vi "DAQmx Create Channel (TEDS-AI-Position-LVDT).vi"(0 "task in":refnum<k21>, 1 "maximum value":dbl=0.1 format="%0.2f", 2 "minimum value":dbl=-0.1 format="%0.2f", 3 "voltage excitation wire mode":i32(ring)=4 items=["4-Wire"=4, "5-Wire"=5, "6-Wire"=6], 5 "physical channels":tag, 6 "voltage excitation source":i32(ring)=10200 items=["Internal"=10200, "External"=10167, "None"=10230], 7 "name to assign":string, 8 "voltage excitation value":dbl=1.0, 9 "units":i32(ring)=10219 items=["Meters"=10219, "Inches"=10379, "From Custom Scale"=10065], 10 "voltage excitation frequency":dbl=2500.0, 11 "error in":errorcluster, 12 "custom scale name":tag) -> (4 "task out":refnum<k21>, 15 "error out":errorcluster)   [LabVIEW 2020]
doc: "Creates channel(s) that use an LVDT to measure linear position. You must configure the physical channel(s) with TEDS information to use this VI."
uses:
  nilvaiu.dll
panel:
  # "input limits"
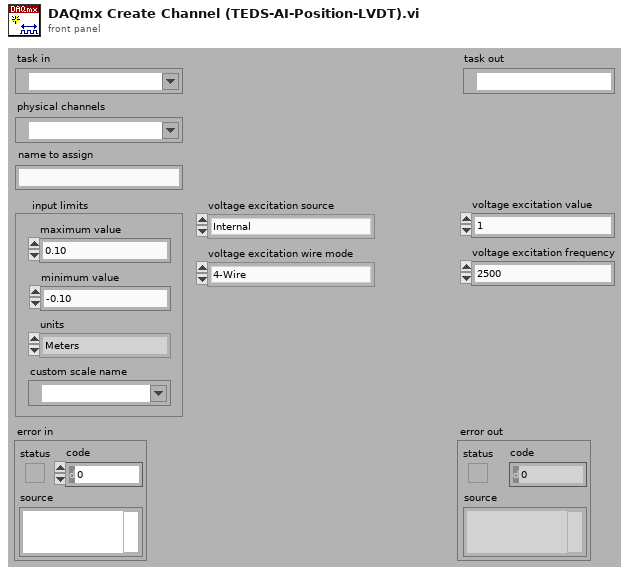
[diagram p1: front panel]
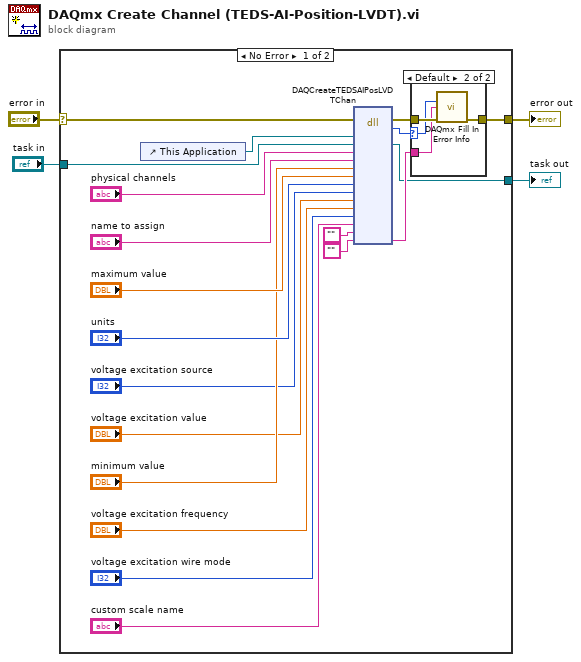
[diagram p0: block diagram]
diagram:
  n1 = case shown="No Error" "error in" {
    selector: "error in" -> [w18 w31]
    tunnel: [w19 w31] -> w2
    tunnel: "task in" -> [w16 w30]
    tunnel: [w17 w30] -> w1
    frame No Error {
      n2 = control-ref of="This Application"() -> (w21:refnum<vi>)
      n3 = dll-call lib="nilvaiu.*" fn="DAQCreateTEDSAIPosLVDTChan"(error in=w18, "lvAppRef"=w21, "refObjPtr"=w16, "physicalChannelName"="physical channels", "channelNameIn"="name to assign", "minVal"="minimum value", "maxVal"="maximum value", "units"="units", "voltageExcitSource"="voltage excitation source", "excitVal"="voltage excitation value", "excitFreq"="voltage excitation frequency", "ACExcitWireMode"="voltage excitation wire mode", "customScaleName"="custom scale name", "channelNamesOut"="", "extendedErrorInfo"="") -> (error out=w24:errorcluster, "return type"=w23:i32, "refObjPtr"=w17:refnum<k21>, "extendedErrorInfo"=w22:string)  [unwired: 14 in, 1 out]
      n4 = case shown="Default" w23 {
        selector: w23 -> [_ w27]
        tunnel: w24 -> [w25 w29]
        tunnel: [w25 w28] -> w19
        tunnel: w22 -> [_ w26]
        frame 0 {
        }
        frame Default {
          n5 = call "DAQmx Fill In Error Info.vi"("status code"=w27, "extended error info"=w26, "error in"=w29) -> ("error out"=w28:errorcluster)  [unwired: 1 in, 11 out]
        }
      }
    }
    frame Error {
    }
  }
  "error out" <- w2
  "task out" <- w1
